vi "coutinuousPathSamplingFPGA4.vi"() -> ()   [LabVIEW 2017]
uses:
  <vilib>/rvi/Emulation/niFpgaSctlEmulationGetInTimedLoop.vi
  <vilib>/rvi/Emulation/niFpgaProcessEmulError.vi
  <vilib>/rvi/interface/RandomDataEmulation/niFpgaRandomDataHandleErrors.vi
  <vilib>/rvi/Emulation/niFpgaGetClockAttributes.vi
  <vilib>/rvi/Emulation/niFpgaEmulationReportErrorSimple.vi
  <vilib>/rvi/eio/common/nirviEmuTemplateMethod_errors.vi
  <vilib>/rvi/Emulation/niFpgaCriticalErrorInLSC.vi
  <vilib>/rvi/DataTransferAndStorage/Container/XNode/niFpgaContainer.xnode
  <vilib>/rvi/interface/RandomDataEmulation/nirviRandomDataFpgaReadWriteTemplate.vi
  <vilib>/eio/EIONode/EIONode.xnode
panel:
  out "y_image_pos_final":u16
  out "x_image_pos_final":u16
  in  "pixel distance":u16
  out "ToRead":u32
  out "increment_x_move":fxp<+/-,55,4>=0.01171875
  out "increment_y_move":fxp<+/-,55,4>=0.01171875
  out "x_FinalPos":fxp<+/-,50,5>
  out "y_FinalPos":fxp<+/-,50,5>
  in  "muPathUpdate Clock (uSec)":fxp<+,32,32>=2400.0
  in  "deflection threshold":fxp<+/-,20,5>=0.0050048828125
  in  "x threshold":fxp<+/-,20,5>=0.0050048828125
  in  "y threshold":fxp<+/-,20,5>=0.0050048828125
  in  "z threshold":fxp<+/-,20,5>=0.0050048828125
  in  "Stage Clock (uSec)":fxp<+,32,32>=500.0
  in  "pixel segment":u32
  out "SettleCheckBuffer":u16=25
  out "a tor buffer":fxp<+,17,1>[](array[numeric])=[1.9999847412109375, 1.9999847412109375, 1.9999847412109375, 1.9999847412109375, 1.9999847412109375, 1.9999847412109375, 1.9999847412109375, 1.9999847412109375, 1.9999847412109375, 1.9999847412109375, 1.9999847412109375, 1.9999847412109375, 1.9999847412109375, 1.9999847412109375, 1.9999847412109375, 1.9999847412109375, 1.9999847412109375, 1.9999847412109375, 1.9999847412109375, 1.9999847412109375, 1.9999847412109375, 1.9999847412109375, 1.9999847412109375, 1.9999847412109375, 1.9999847412109375]
  out "b tor buffer":fxp<+,17,1>[](array[numeric])=[1.9999847412109375, 1.9999847412109375, 1.9999847412109375, 1.9999847412109375, 1.9999847412109375, 1.9999847412109375, 1.9999847412109375, 1.9999847412109375, 1.9999847412109375, 1.9999847412109375, 1.9999847412109375, 1.9999847412109375, 1.9999847412109375, 1.9999847412109375, 1.9999847412109375, 1.9999847412109375, 1.9999847412109375, 1.9999847412109375, 1.9999847412109375, 1.9999847412109375, 1.9999847412109375, 1.9999847412109375, 1.9999847412109375, 1.9999847412109375, 1.9999847412109375]
  in  "deflection control":T1={"SetPoint (V)"=0.0, "scanning I"=0.03125, "scanning P"=0.0498046875, "Initial I (V)"=0.0, "Upper Limit (V)"=8.0, "Lower Limit (V)"=-8.0}
  out "deflection sensor":fxp<+/-,20,5>=-0.271331787109375
  out "zControlMode":bool
  in  "Z Clock (uSec)":fxp<+,32,32>=10.0
  out "stageIndicator":u8=1
  in  "z control":T2={"SetPoint (V)"=-0.19999980926513672, "I"=0.03125, "P"=0.0498046875, "Initial I (V)"=0.0, "Upper Limit (V)"=8.0, "Lower Limit (V)"=-8.0}
  out "signalToRecord":bool
  out "z output":fxp<+/-,64,29>=-3.5890110712498426
  in  "Sampling Clock (uSec)":fxp<+,32,32>=1500.0
  out "x output":fxp<+/-,64,29>=0.00029289722442626953
  out "y output":fxp<+/-,64,29>=0.29396580904722214
  out "x sensor":fxp<+/-,20,5>
  out "y sensor":fxp<+/-,20,5>=-0.285125732421875
  in  "XY Clock (uSec)":fxp<+,32,32>=50.0
  in  "y control":T1={"SetPoint (V)"=0.0, "scanning I"=0.03125, "scanning P"=0.0498046875, "Initial I (V)"=0.0, "Upper Limit (V)"=8.0, "Lower Limit (V)"=-8.0}
  in  "x control":T1={"SetPoint (V)"=0.0, "scanning I"=0.03125, "scanning P"=0.0498046875, "Initial I (V)"=0.0, "Upper Limit (V)"=8.0, "Lower Limit (V)"=-8.0}
  out "signalToStop":bool
  out "x_pos":fxp<+/-,50,5>=0.005859375
  out "y_pos":fxp<+/-,50,5>=0.005859375
  out "increment_x":fxp<+/-,50,5>=0.01171875
  out "increment_y":fxp<+/-,50,5>=0.01171875
  in  "ImageToSample":T3={"image size_x"=256, "image size_y"=256, "sample start_x"=0.0, "sample start_y"=0.0, "sample end_x"=3.0, "sample end_y"=3.0}
  out "y_image_pos":u16
  out "x_image_pos":u16
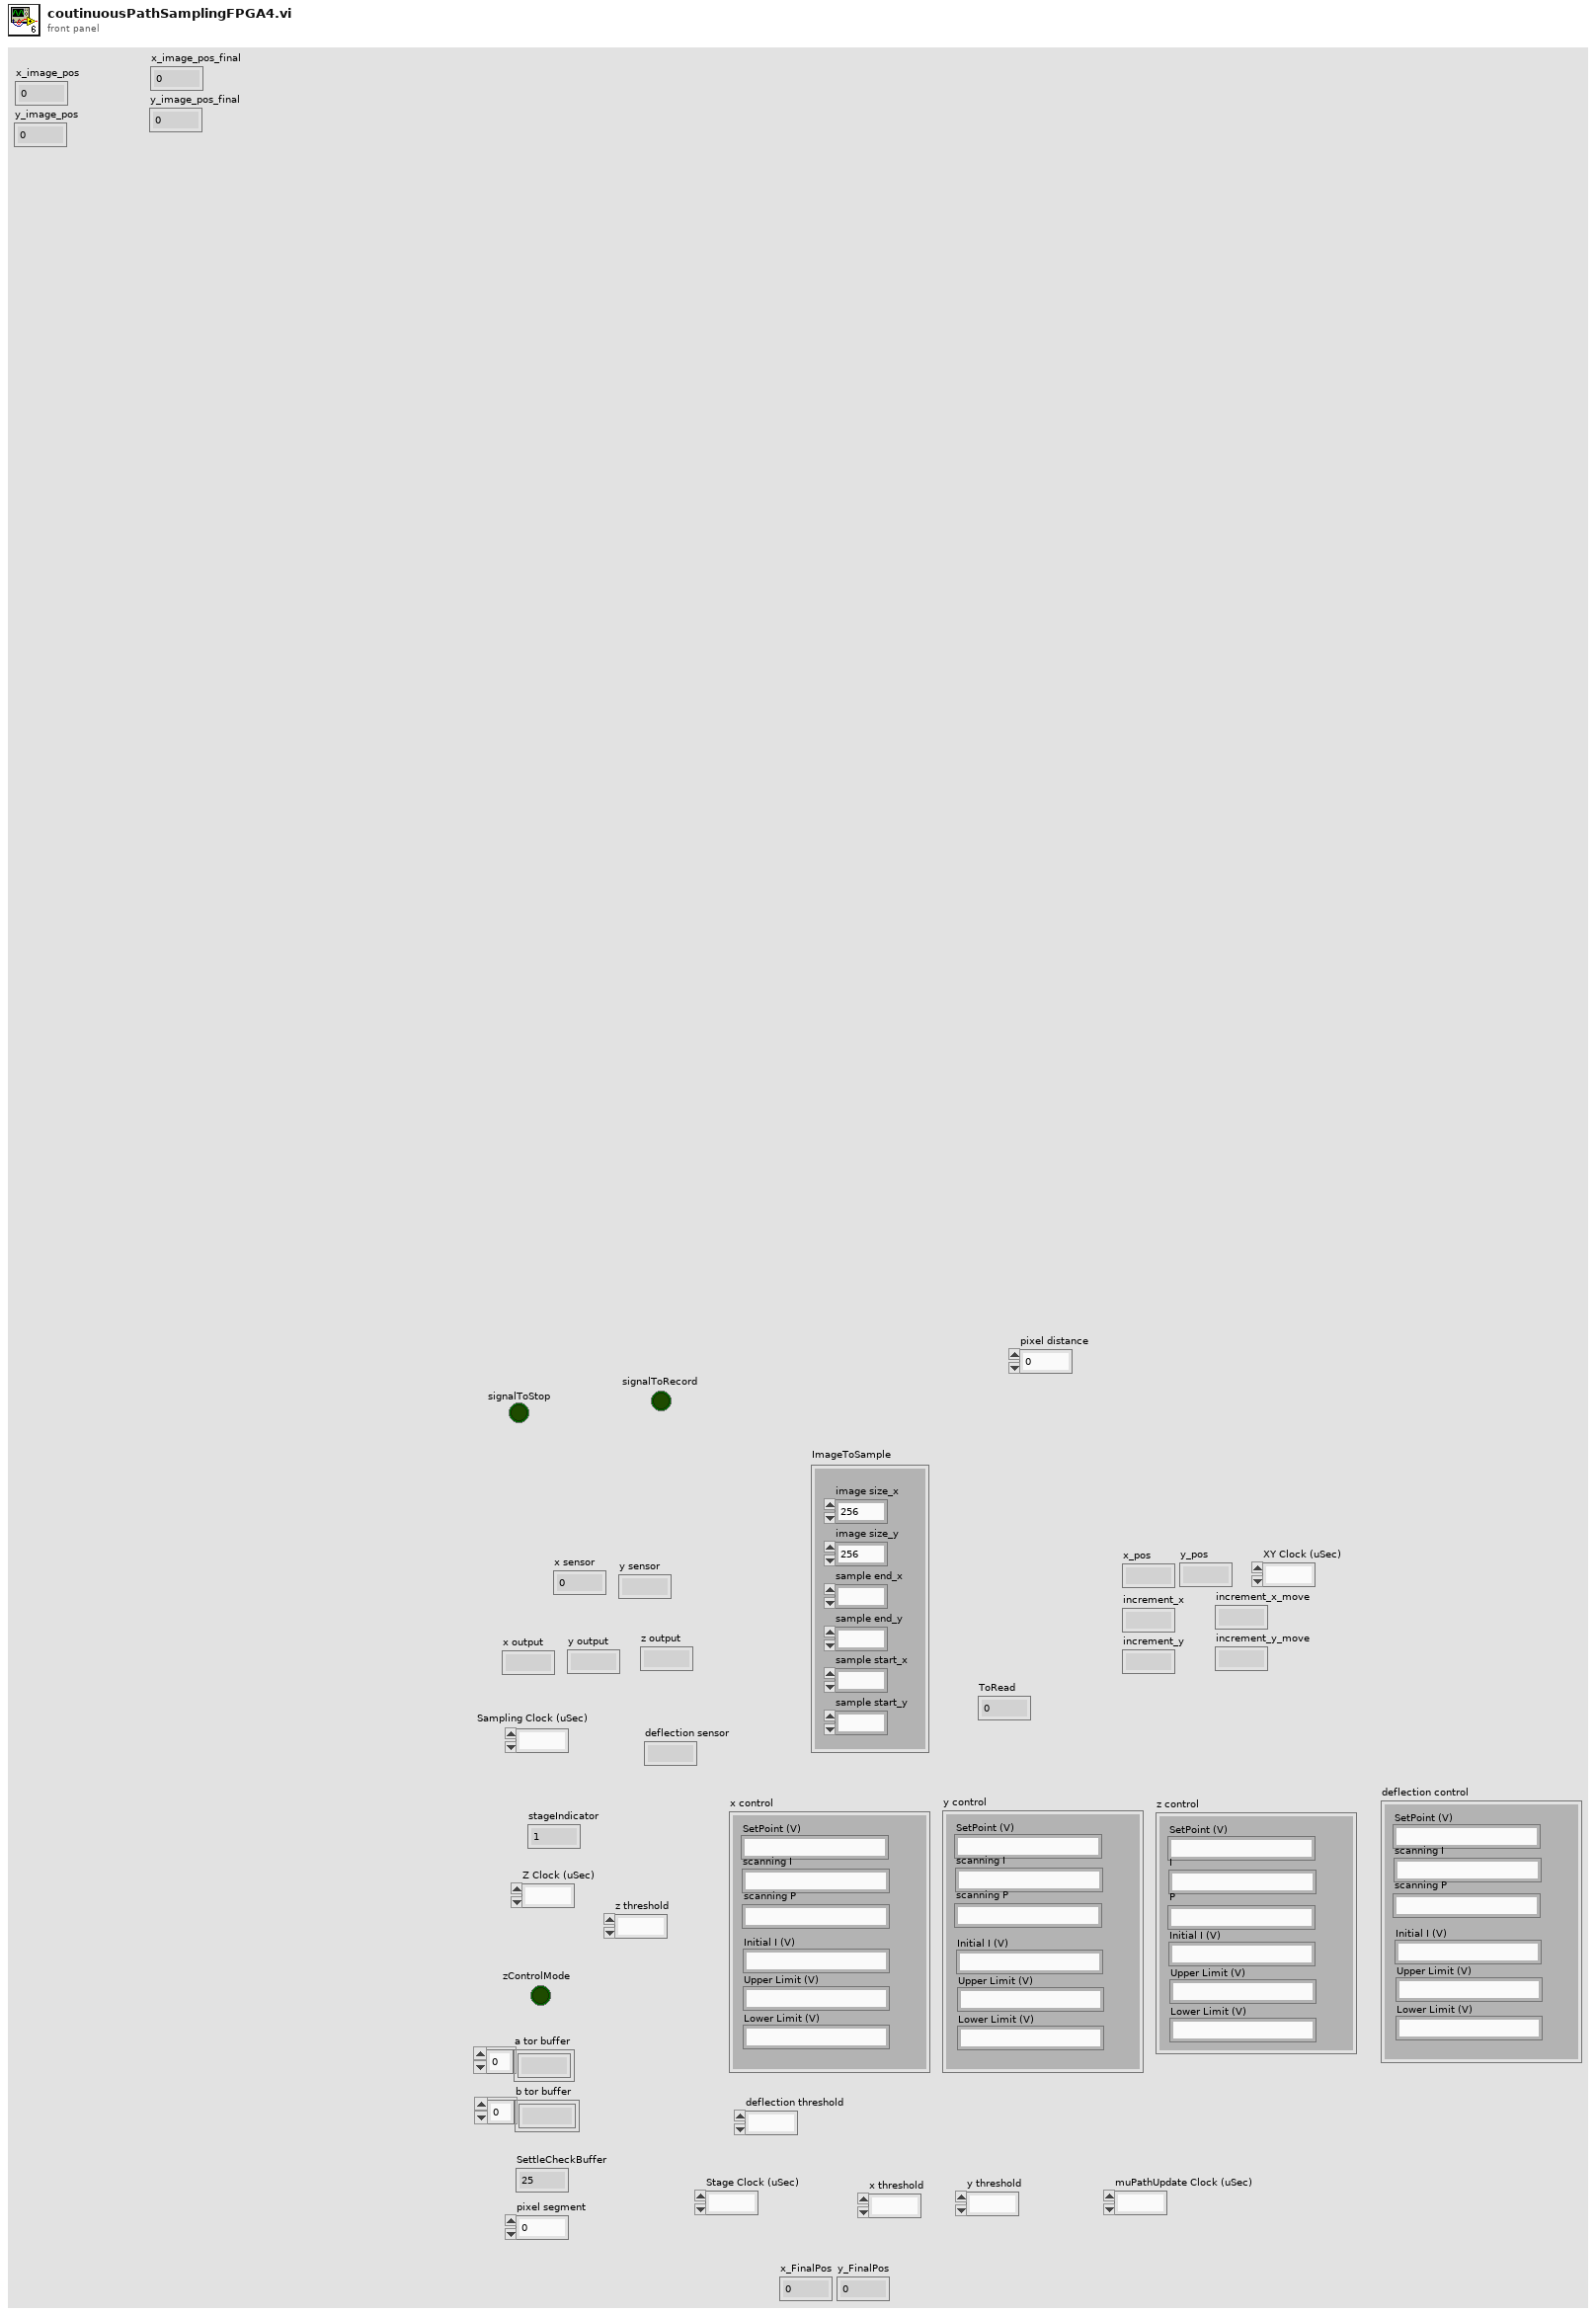
[diagram p1: front panel]
types:
  T1 = cluster{"SetPoint (V)":fxp<+/-,26,5>, "scanning I":fxp<+,21,13>, "scanning P":fxp<+,15,5>, "Initial I (V)":fxp<+/-,10,5>, "Upper Limit (V)":fxp<+/-,26,5>, "Lower Limit (V)":fxp<+/-,26,5>}
  T2 = cluster{"SetPoint (V)":fxp<+/-,26,5>, "I":fxp<+,21,13>, "P":fxp<+,15,5>, "Initial I (V)":fxp<+/-,10,5>, "Upper Limit (V)":fxp<+/-,26,5>, "Lower Limit (V)":fxp<+/-,26,5>}
  T3 = cluster{"image size_x":u16, "image size_y":u16, "sample start_x":fxp<+/-,26,5>, "sample start_y":fxp<+/-,26,5>, "sample end_x":fxp<+/-,26,5>, "sample end_y":fxp<+/-,26,5>}
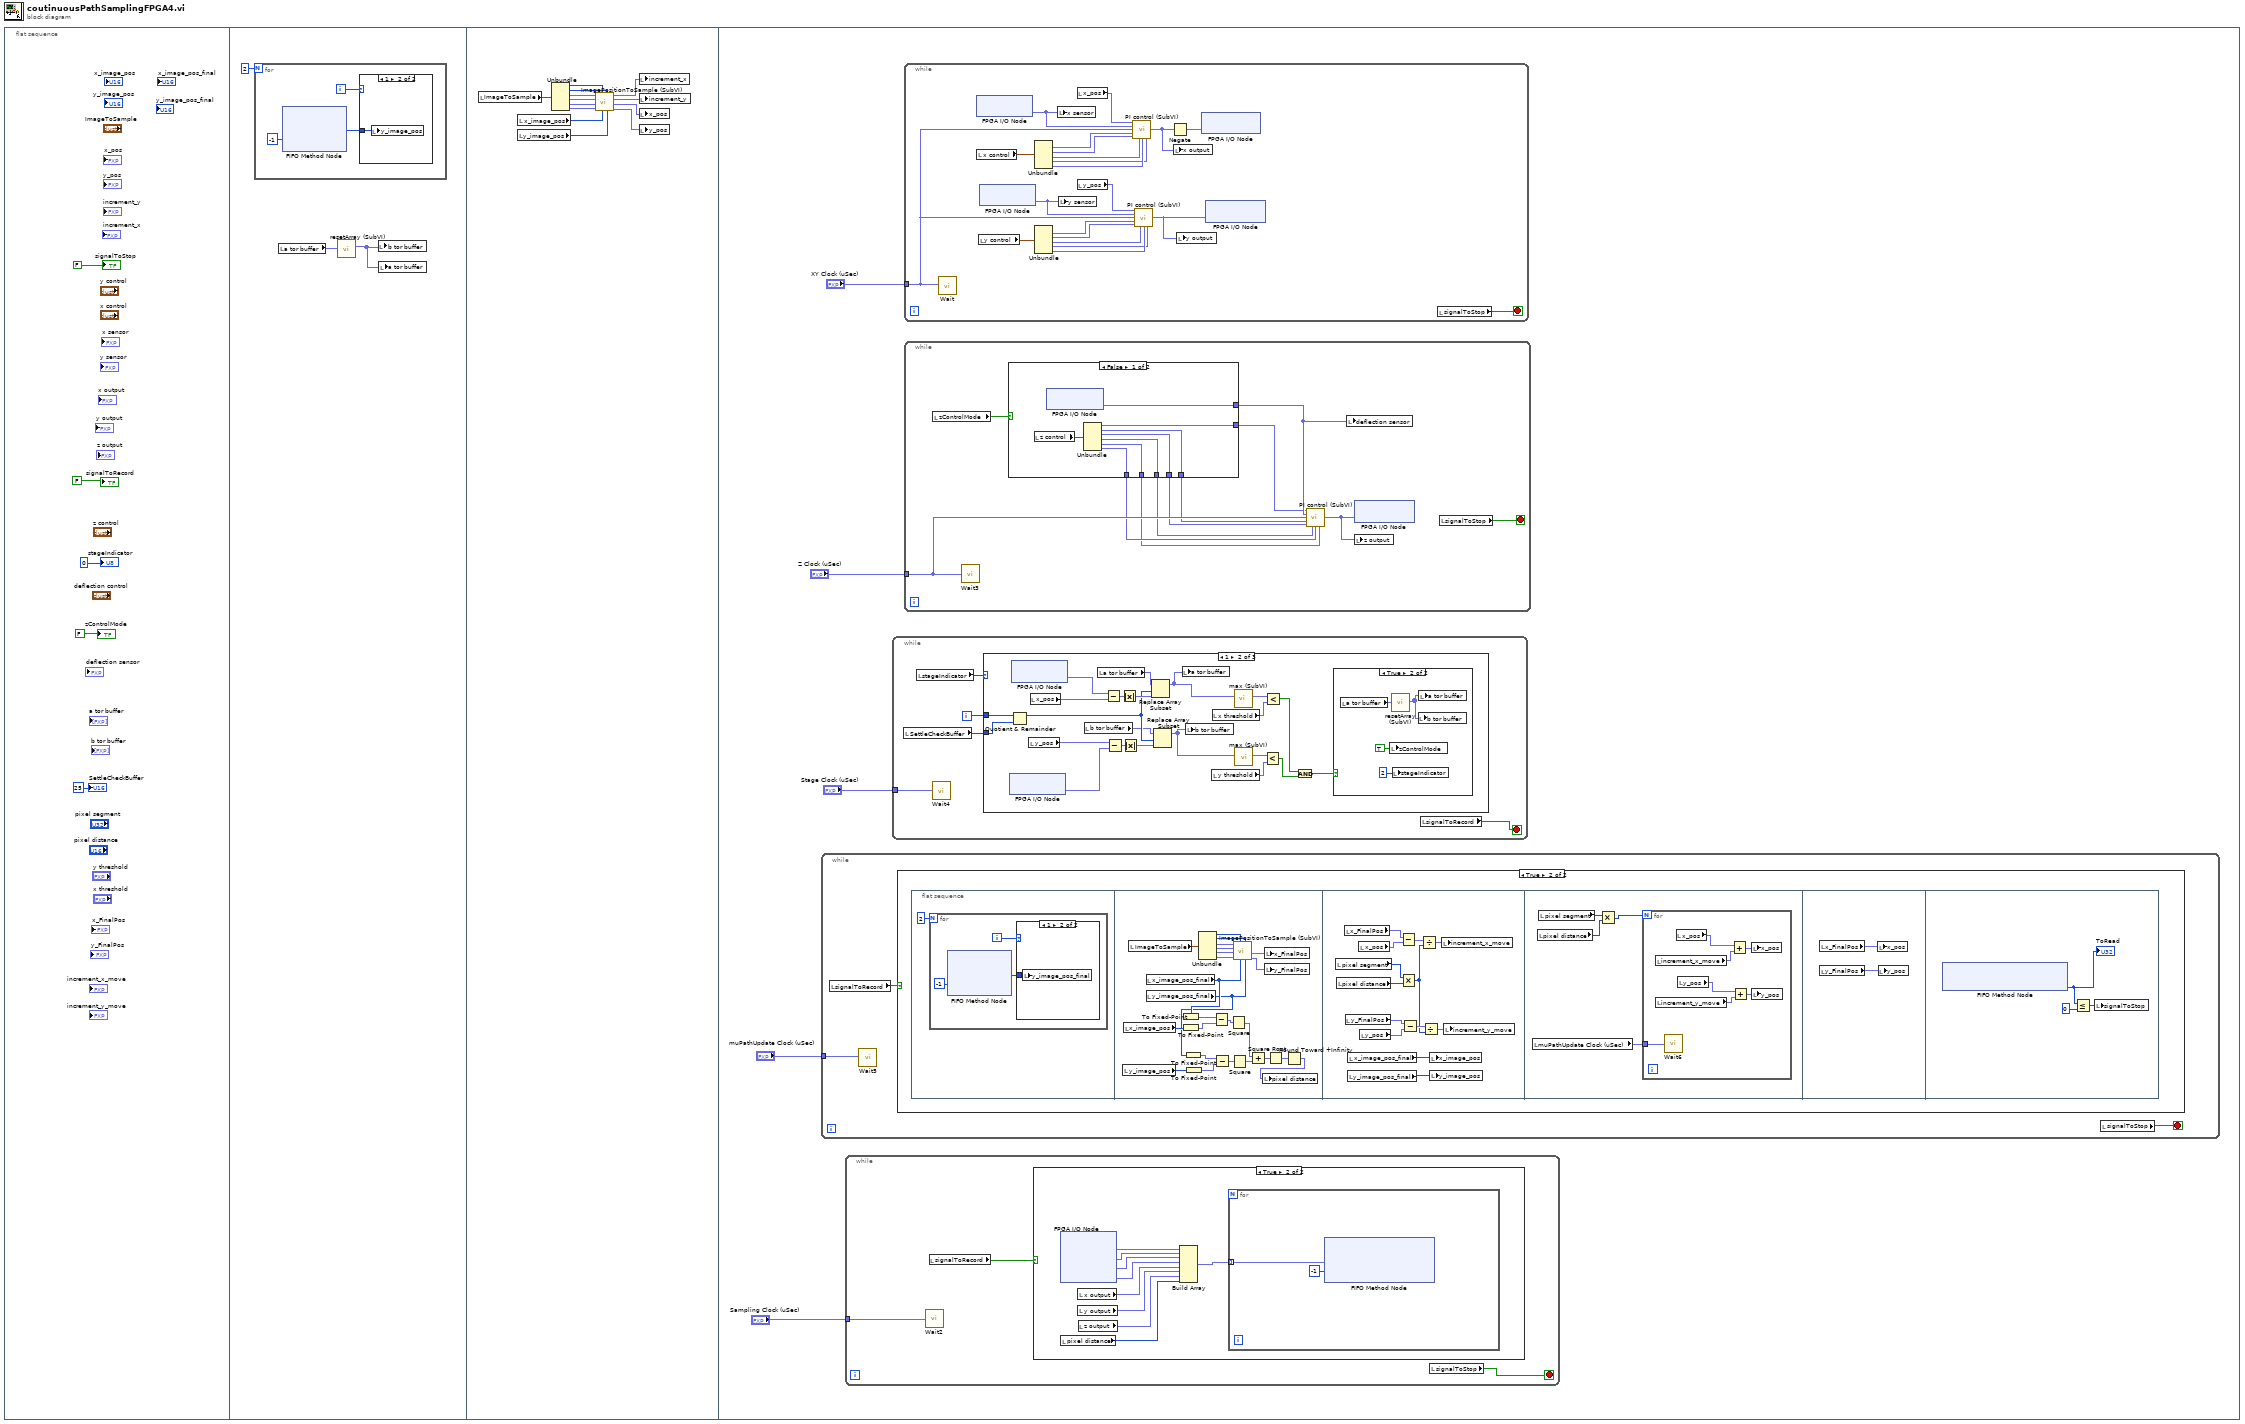
[diagram p0: block diagram]
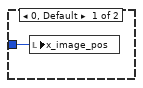
[diagram p2: hidden frame]
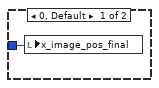
[diagram p4: hidden frame]
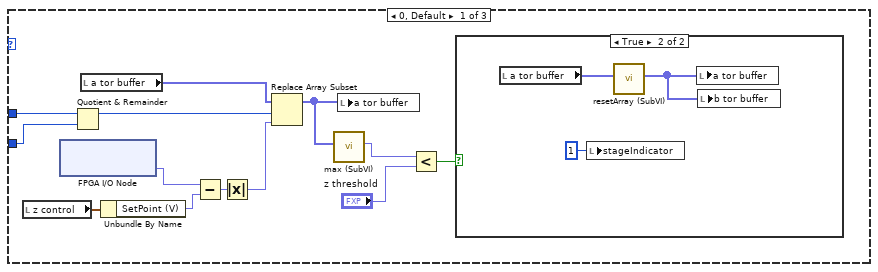
[diagram p5: hidden frame]
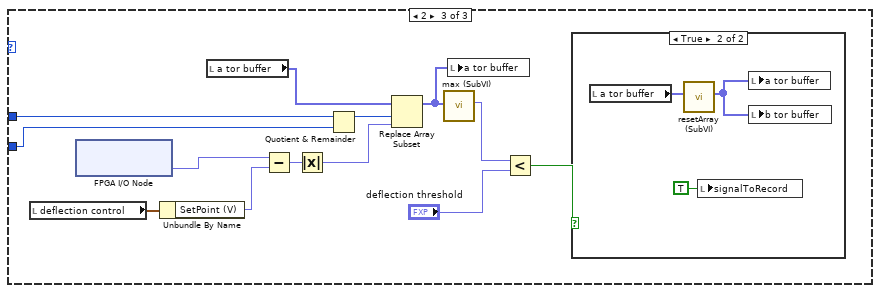
[diagram p8: hidden frame]
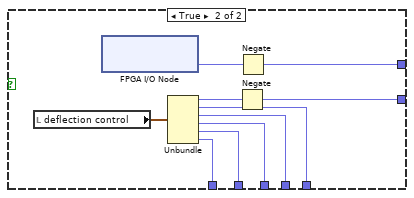
[diagram p10: hidden frame]
diagram:
  n1 = flat-sequence {
    frame #0 {
      "signalToStop" <- FALSE ("signalToStop")
      "signalToRecord" <- FALSE ("signalToRecord")
      "stageIndicator" <- u8 0 ("stageIndicator")
      "zControlMode" <- FALSE ("zControlMode")
      "SettleCheckBuffer" <- u16 25 ("SettleCheckBuffer")
    }
    frame #1 {
      n2 = for {
        N: 2 -> [_]
        i -> [w10]
        n3 = xnode ("FIFO Method Node")("Timeout"=-1) -> ("Element"=w9:u16)  [unwired: 1 in, 2 out]
        n4 = case shown="1" w10 {
          tunnel: w9 -> [w12 w13]
          frame 0, Default {
            n5 = local write "x_image_pos"(w12) -> ()
          }
          frame 1 {
            n6 = local write "y_image_pos"(w13) -> ()
          }
        }
      }
      n7 = local read "a tor buffer"() -> (w7:fxp<+,17,1>[])
      n8 = call "resetArray (SubVI).vi"("a samples in"=w7) -> ("a samples out"=w6:fxp<+/-,64,32>[])  [unwired: 10 in]
      n9 = local write "b tor buffer"(w6) -> ()
      n10 = local write "a tor buffer"(w6) -> ()
    }
    frame #2 {
      n11 = local read "ImageToSample"() -> (w26:T3)
      n12 = local read "y_image_pos"() -> (w18:u16)
      n13 = local read "x_image_pos"() -> (w19:u16)
      n14 = Unbundle(w26) -> ("image size_x"=w25:u16, "image size_y"=w24:u16, "sample start_x"=w23:fxp<+/-,26,5>, "sample start_y"=w22:fxp<+/-,26,5>, "sample end_x"=w21:fxp<+/-,26,5>, "sample end_y"=w20:fxp<+/-,26,5>)
      n15 = call "ImagePositionToSample (SubVI).vi"("image_y"=w18, "image size_y"=w24, "image_x"=w19, "image size_x"=w25, "sample end_y"=w20, "sample end_x"=w21, "sample start_y"=w22, "sample start_x"=w23) -> ("sample_y"=w14:fxp<+/-,26,5>, "sample_x"=w15:fxp<+/-,26,5>, "increment_y"=w16:fxp<+/-,26,5>, "increment_x"=w17:fxp<+/-,26,5>)
      n16 = local write "increment_x"(w17) -> ()
      n17 = local write "increment_y"(w16) -> ()
      n18 = local write "x_pos"(w15) -> ()
      n19 = local write "y_pos"(w14) -> ()
    }
    frame #3 {
      n20 = while {
        tunnel: "muPathUpdate Clock (uSec)" -> [w33]
        stop <- w34 stop-if-true
        n21 = local read "signalToRecord"() -> (w32:bool)
        n22 = call "Wait5"("Count(uSec)"=w33) -> ()  [unwired: 1 out]
        n23 = case shown="True" w32 {
          frame False {
          }
          frame True {
            n24 = flat-sequence {
              frame #0 {
                n25 = for {
                  N: 2 -> [_]
                  i -> [w37]
                  n26 = xnode ("FIFO Method Node")("Timeout"=-1) -> ("Element"=w36:u16)  [unwired: 1 in, 2 out]
                  n27 = case shown="1" w37 {
                    tunnel: w36 -> [w39 w40]
                    frame 0, Default {
                      n28 = local write "x_image_pos_final"(w39) -> ()
                    }
                    frame 1 {
                      n29 = local write "y_image_pos_final"(w40) -> ()
                    }
                  }
                }
              }
              frame #1 {
                n30 = local read "y_image_pos"() -> (w46:u16)
                n31 = local read "x_image_pos"() -> (w47:u16)
                n32 = local read "ImageToSample"() -> (w64:T3)
                n33 = local read "x_image_pos_final"() -> (w50:u16)
                n34 = local read "y_image_pos_final"() -> (w43:u16)
                n35 = To Fixed-Point(number=w50) -> (fixed-point=w49:fxp<+,16,16>)  [unwired: 1 in]
                n36 = To Fixed-Point(number=w47) -> (fixed-point=w48:fxp<+,16,16>)  [unwired: 1 in]
                n37 = To Fixed-Point(number=w43) -> (fixed-point=w44:fxp<+,16,16>)  [unwired: 1 in]
                n38 = To Fixed-Point(number=w46) -> (fixed-point=w45:fxp<+,16,16>)  [unwired: 1 in]
                n39 = Unbundle(w64) -> ("image size_x"=w63:u16, "image size_y"=w62:u16, "sample start_x"=w61:fxp<+/-,26,5>, "sample start_y"=w60:fxp<+/-,26,5>, "sample end_x"=w59:fxp<+/-,26,5>, "sample end_y"=w58:fxp<+/-,26,5>)
                n40 = Subtract(x=w49, y=w48) -> (x-y=w52:fxp<+/-,17,17>)
                n41 = Subtract(x=w44, y=w45) -> (x-y=w51:fxp<+/-,17,17>)
                n42 = Square(x=w52) -> (x^2=w54:fxp<+,32,32>)
                n43 = Square(x=w51) -> (x^2=w55:fxp<+,32,32>)
                n44 = call "ImagePositionToSample (SubVI).vi"("image_y"=w43, "image size_y"=w62, "image_x"=w50, "image size_x"=w63, "sample end_y"=w58, "sample end_x"=w59, "sample start_y"=w60, "sample start_x"=w61) -> ("sample_y"=w56:fxp<+/-,26,5>, "sample_x"=w57:fxp<+/-,26,5>)  [unwired: 2 out]
                n45 = Add(x=w54, y=w55) -> (x+y=w53:fxp<+,33,33>)
                n46 = local write "x_FinalPos"(w57) -> ()
                n47 = local write "y_FinalPos"(w56) -> ()
                n48 = Square Root(x=w53) -> (sqrt(x)=w42:fxp<+,36,17>)
                n49 = Round Toward +Infinity(x=w42) -> (ceil(x): smallest int >= x=w41:fxp<+,17,17>)
                n50 = local write "pixel distance"(w41) -> ()
              }
              frame #2 {
                n51 = local read "pixel segment"() -> (w68:u32)
                n52 = local read "pixel distance"() -> (w67:u16)
                n53 = local read "x_FinalPos"() -> (w77:fxp<+/-,50,5>)
                n54 = local read "y_FinalPos"() -> (w71:fxp<+/-,50,5>)
                n55 = local read "y_image_pos_final"() -> (w65:u16)
                n56 = local read "x_image_pos_final"() -> (w66:u16)
                n57 = local read "x_pos"() -> (w76:fxp<+/-,50,5>)
                n58 = local read "y_pos"() -> (w70:fxp<+/-,50,5>)
                n59 = Subtract(x=w77, y=w76) -> (x-y=w75:fxp<+/-,51,6>)
                n60 = Multiply(x=w68, y=w67) -> (x*y=w69:u32)
                n61 = Subtract(x=w71, y=w70) -> (x-y=w73:fxp<+/-,51,6>)
                n62 = Divide(x=w75, y=w69) -> (x/y=w74:fxp<+/-,64,6>)
                n63 = Divide(x=w73, y=w69) -> (x/y=w72:fxp<+/-,64,6>)
                n64 = local write "x_image_pos"(w66) -> ()
                n65 = local write "y_image_pos"(w65) -> ()
                n66 = local write "increment_x_move"(w74) -> ()
                n67 = local write "increment_y_move"(w72) -> ()
              }
              frame #3 {
                n68 = local read "muPathUpdate Clock (uSec)"() -> (w81:fxp<+,32,32>)
                n69 = local read "pixel distance"() -> (w78:u16)
                n70 = local read "pixel segment"() -> (w80:u32)
                n71 = Multiply(x=w80, y=w78) -> (x*y=w79:u32)
                n72 = for {
                  N: w79 -> [_]
                  tunnel: w81 -> [w88]
                  n73 = local read "increment_x_move"() -> (w86:fxp<+/-,55,4>)
                  n74 = local read "increment_y_move"() -> (w83:fxp<+/-,55,4>)
                  n75 = call "Wait6"("Count(uSec)"=w88) -> ()  [unwired: 1 out]
                  n76 = local read "x_pos"() -> (w87:fxp<+/-,50,5>)
                  n77 = local read "y_pos"() -> (w84:fxp<+/-,50,5>)
                  n78 = Add(x=w87, y=w86) -> (x+y=w85:fxp<+/-,57,6>)
                  n79 = Add(x=w84, y=w83) -> (x+y=w82:fxp<+/-,57,6>)
                  n80 = local write "x_pos"(w85) -> ()
                  n81 = local write "y_pos"(w82) -> ()
                }
              }
              frame #4 {
                n82 = local read "x_FinalPos"() -> (w90:fxp<+/-,50,5>)
                n83 = local read "y_FinalPos"() -> (w89:fxp<+/-,50,5>)
                n84 = local write "x_pos"(w90) -> ()
                n85 = local write "y_pos"(w89) -> ()
              }
              frame #5 {
                n86 = xnode ("FIFO Method Node")() -> ("Number of Elements to Read"=w91:u32)  [unwired: 1 in, 1 out]
                "ToRead" <- w91
                n87 = Less Or Equal?(x=w91, y=u32 0) -> (x <= y?=w92:bool)
                n88 = local write "signalToStop"(w92) -> ()
              }
            }
          }
        }
        n89 = local read "signalToStop"() -> (w34:bool)
      }
      n90 = while {
        tunnel: "Sampling Clock (uSec)" -> [w188]
        stop <- w187 stop-if-true
        n91 = call "Wait2"("Count(uSec)"=w188) -> ()  [unwired: 1 out]
        n92 = local read "signalToRecord"() -> (w186:bool)
        n93 = case shown="True" w186 {
          frame False {
          }
          frame True {
            n94 = xnode "FPGA I/O Node"() -> ("Mod1/AI0"=w197:fxp<+/-,20,5>, "Mod1/AI1"=w196:fxp<+/-,20,5>, "Mod1/AI2"=w195:fxp<+/-,20,5>, "Mod1/AI3"=w194:fxp<+/-,20,5>)  [unwired: 4 in, 4 out]
            n95 = local read "pixel distance"() -> (w189:u16)
            n96 = local read "x output"() -> (w193:fxp<+/-,64,29>)
            n97 = local read "y output"() -> (w192:fxp<+/-,64,29>)
            n98 = local read "z output"() -> (w191:fxp<+/-,64,29>)
            n99 = Build Array(w197, w196, w195, w194, w193, w192, w191, w189) -> (w190:fxp<+/-,64,29>[])
            n100 = for {
              tunnel: w190 -> [w199] mode=indexing
              n101 = xnode ("FIFO Method Node")("Element"=w199, "Timeout"=-1) -> ()  [unwired: 1 in, 2 out]
            }
          }
        }
        n102 = local read "signalToStop"() -> (w187:bool)
      }
      n103 = while {
        tunnel: "Stage Clock (uSec)" -> [w98]
        i -> [w96]
        stop <- w94 stop-if-true
        n104 = local read "SettleCheckBuffer"() -> (w95:u16)
        n105 = local read "stageIndicator"() -> (w97:u8)
        n106 = call "Wait4"("Count(uSec)"=w98) -> ()  [unwired: 1 out]
        n107 = case shown="1" w97 {
          tunnel: w96 -> [w111 w136 w153]
          tunnel: w95 -> [w110 w135 w152]
          frame 0, Default {
            n108 = local read "z control"() -> (w104:T2)
            n109 = xnode "FPGA I/O Node"() -> ("Mod1/AI2"=w106:fxp<+/-,20,5>)  [unwired: 1 in, 1 out]
            n110 = Quotient & Remainder(x=w111, y=w110) -> (x-y*floor(x/y)=w109:i32)  [unwired: 1 out]
            n111 = local read "a tor buffer"() -> (w105:fxp<+,17,1>[])
            n112 = Unbundle By Name(w104) -> ("SetPoint (V)"=w103:fxp<+/-,26,5>)
            n113 = Subtract(x=w106, y=w103) -> (x-y=w108:fxp<+/-,27,6>)
            n114 = Absolute Value(x=w108) -> (abs(x)=w107:fxp<+,26,5>)
            n115 = Replace Array Subset(array=w105, new element=w107, index=w109) -> (w102:fxp<+,17,1>[])
            n116 = call "max (SubVI).vi"("initialized array"=w102) -> ("y"=w101:fxp<+/-,64,32>)  [unwired: 10 in]
            n117 = local write "a tor buffer"(w102) -> ()
            n118 = Less?(x=w101, y="z threshold") -> (x < y?=w99:bool)
            n119 = case shown="True" w99 {
              frame False {
              }
              frame True {
                n120 = local read "a tor buffer"() -> (w114:fxp<+,17,1>[])
                n121 = local write "stageIndicator"(u8 1 ("stageIndicator")) -> ()
                n122 = call "resetArray (SubVI).vi"("a samples in"=w114) -> ("a samples out"=w113:fxp<+/-,64,32>[])  [unwired: 10 in]
                n123 = local write "a tor buffer"(w113) -> ()
                n124 = local write "b tor buffer"(w113) -> ()
              }
            }
          }
          frame 1 {
            n125 = xnode "FPGA I/O Node"() -> ("Mod1/AI1"=w117:fxp<+/-,20,5>)  [unwired: 1 in, 1 out]
            n126 = Quotient & Remainder(x=w136, y=w135) -> (x-y*floor(x/y)=w127:i32)  [unwired: 1 out]
            n127 = xnode "FPGA I/O Node"() -> ("Mod1/AI0"=w118:fxp<+/-,20,5>)  [unwired: 1 in, 1 out]
            n128 = local read "y_pos"() -> (w115:fxp<+/-,50,5>)
            n129 = local read "x_pos"() -> (w116:fxp<+/-,50,5>)
            n130 = local read "b tor buffer"() -> (w125:fxp<+,17,1>[])
            n131 = local read "a tor buffer"() -> (w126:fxp<+,17,1>[])
            n132 = Subtract(x=w118, y=w116) -> (x-y=w131:fxp<+/-,51,6>)
            n133 = Subtract(x=w115, y=w117) -> (x-y=w129:fxp<+/-,51,6>)
            n134 = Absolute Value(x=w131) -> (abs(x)=w130:fxp<+,50,5>)
            n135 = Absolute Value(x=w129) -> (abs(x)=w128:fxp<+,50,5>)
            n136 = Replace Array Subset(array=w126, new element=w130, index=w127) -> (w124:fxp<+,17,1>[])
            n137 = Replace Array Subset(array=w125, new element=w128, index=w127) -> (w123:fxp<+,17,1>[])
            n138 = local write "a tor buffer"(w124) -> ()
            n139 = local write "b tor buffer"(w123) -> ()
            n140 = local read "y threshold"() -> (w119:fxp<+/-,20,5>)
            n141 = local read "x threshold"() -> (w121:fxp<+/-,20,5>)
            n142 = call "max (SubVI).vi"("initialized array"=w124) -> ("y"=w122:fxp<+/-,64,32>)  [unwired: 10 in]
            n143 = call "max (SubVI).vi"("initialized array"=w123) -> ("y"=w120:fxp<+/-,64,32>)  [unwired: 10 in]
            n144 = Less?(x=w120, y=w119) -> (x < y?=w133:bool)
            n145 = Less?(x=w122, y=w121) -> (x < y?=w134:bool)
            n146 = And(x=w134, y=w133) -> (x .and. y?=w132:bool)
            n147 = case shown="True" w132 {
              frame False {
              }
              frame True {
                n148 = local read "a tor buffer"() -> (w139:fxp<+,17,1>[])
                n149 = local write "zControlMode"(TRUE ("zControlMode")) -> ()
                n150 = call "resetArray (SubVI).vi"("a samples in"=w139) -> ("a samples out"=w138:fxp<+/-,64,32>[])  [unwired: 10 in]
                n151 = local write "stageIndicator"(u8 2 ("stageIndicator")) -> ()
                n152 = local write "b tor buffer"(w138) -> ()
                n153 = local write "a tor buffer"(w138) -> ()
              }
            }
          }
          frame 2 {
            n154 = local read "deflection control"() -> (w149:T1)
            n155 = xnode "FPGA I/O Node"() -> ("Mod1/AI3"=w147:fxp<+/-,20,5>)  [unwired: 1 in, 1 out]
            n156 = Unbundle By Name(w149) -> ("SetPoint (V)"=w148:fxp<+/-,26,5>)
            n157 = local read "a tor buffer"() -> (w143:fxp<+,17,1>[])
            n158 = Subtract(x=w147, y=w148) -> (x-y=w151:fxp<+/-,27,6>)
            n159 = Absolute Value(x=w151) -> (abs(x)=w146:fxp<+,26,5>)
            n160 = Quotient & Remainder(x=w153, y=w152) -> (x-y*floor(x/y)=w150:i32)  [unwired: 1 out]
            n161 = Replace Array Subset(array=w143, new element=w146, index=w150) -> (w142:fxp<+,17,1>[])
            n162 = call "max (SubVI).vi"("initialized array"=w142) -> ("y"=w145:fxp<+/-,64,32>)  [unwired: 10 in]
            n163 = local write "a tor buffer"(w142) -> ()
            n164 = Less?(x=w145, y="deflection threshold") -> (x < y?=w141:bool)
            n165 = case shown="True" w141 {
              frame False {
              }
              frame True {
                n166 = local read "a tor buffer"() -> (w156:fxp<+,17,1>[])
                n167 = call "resetArray (SubVI).vi"("a samples in"=w156) -> ("a samples out"=w155:fxp<+/-,64,32>[])  [unwired: 10 in]
                n168 = local write "signalToRecord"(TRUE ("signalToRecord")) -> ()
                n169 = local write "a tor buffer"(w155) -> ()
                n170 = local write "b tor buffer"(w155) -> ()
              }
            }
          }
        }
        n171 = local read "signalToRecord"() -> (w94:bool)
      }
      n172 = while {
        tunnel: "XY Clock (uSec)" -> [w206]
        stop <- w220 stop-if-true
        n173 = call "Wait"("Count(uSec)"=w206) -> ()  [unwired: 1 out]
        n174 = xnode "FPGA I/O Node"() -> ("Mod1/AI0"=w217:fxp<+/-,20,5>)  [unwired: 1 in, 1 out]
        n175 = local read "x control"() -> (w219:T1)
        n176 = local read "y control"() -> (w207:T1)
        n177 = xnode "FPGA I/O Node"() -> ("Mod1/AI1"=w208:fxp<+/-,20,5>)  [unwired: 1 in, 1 out]
        n178 = Unbundle(w219) -> ("scanning I"=w216:fxp<+,21,13>, "scanning P"=w215:fxp<+,15,5>, "Initial I (V)"=w214:fxp<+/-,10,5>, "Upper Limit (V)"=w212:fxp<+/-,26,5>, "Lower Limit (V)"=w213:fxp<+/-,26,5>)  [unwired: 1 out]
        n179 = Unbundle(w207) -> ("scanning I"=w205:fxp<+,21,13>, "scanning P"=w204:fxp<+,15,5>, "Initial I (V)"=w203:fxp<+/-,10,5>, "Upper Limit (V)"=w201:fxp<+/-,26,5>, "Lower Limit (V)"=w202:fxp<+/-,26,5>)  [unwired: 1 out]
        n180 = local write "x sensor"(w217) -> ()
        n181 = local write "y sensor"(w208) -> ()
        n182 = local read "x_pos"() -> (w218:fxp<+/-,50,5>)
        n183 = local read "y_pos"() -> (w209:fxp<+/-,50,5>)
        n184 = call "PI control (SubVI).vi"("SetPoint"=w218, "Feedback"=w217, "Clock"=w206, "I"=w216, "P"=w215, "Initial I"=w214, "Lower Limit"=w213, "Upper Limit in"=w212) -> ("Output"=w211:fxp<+/-,20,5>)  [unwired: 7 in]
        n185 = call "PI control (SubVI).vi"("SetPoint"=w209, "Feedback"=w208, "Clock"=w206, "I"=w205, "P"=w204, "Initial I"=w203, "Lower Limit"=w202, "Upper Limit in"=w201) -> ("Output"=w200:fxp<+/-,20,5>)  [unwired: 7 in]
        n186 = Negate(x=w211) -> (-x=w210:fxp<+/-,21,6>)
        n187 = local write "x output"(w211) -> ()
        n188 = local write "y output"(w200) -> ()
        n189 = xnode "FPGA I/O Node"("Mod8/AO0"=w210) -> ()  [unwired: 1 in, 1 out]
        n190 = xnode "FPGA I/O Node"("Mod8/AO1"=w200) -> ()  [unwired: 1 in, 1 out]
        n191 = local read "signalToStop"() -> (w220:bool)
      }
      n192 = while {
        tunnel: "Z Clock (uSec)" -> [w162]
        stop <- w167 stop-if-true
        n193 = local read "zControlMode"() -> (w166:bool)
        n194 = call "Wait3"("Count(uSec)"=w162) -> ()  [unwired: 1 out]
        n195 = case shown="False" w166 {
          tunnel: [w174 w183] -> w164
          tunnel: [w173 w181] -> w163
          tunnel: [w172 w180] -> w161
          tunnel: [w171 w179] -> w160
          tunnel: [w170 w178] -> w159
          tunnel: [w169 w177] -> w158
          tunnel: [w168 w176] -> w157
          frame False {
            n196 = local read "z control"() -> (w175:T2)
            n197 = xnode "FPGA I/O Node"() -> ("Mod1/AI2"=w174:fxp<+/-,20,5>)  [unwired: 1 in, 1 out]
            n198 = Unbundle(w175) -> ("SetPoint (V)"=w173:fxp<+/-,26,5>, "I"=w172:fxp<+,21,13>, "P"=w171:fxp<+,15,5>, "Initial I (V)"=w170:fxp<+/-,10,5>, "Upper Limit (V)"=w168:fxp<+/-,26,5>, "Lower Limit (V)"=w169:fxp<+/-,26,5>)
          }
          frame True {
            n199 = local read "deflection control"() -> (w185:T1)
            n200 = xnode "FPGA I/O Node"() -> ("Mod1/AI3"=w184:fxp<+/-,20,5>)  [unwired: 1 in, 1 out]
            n201 = Unbundle(w185) -> ("SetPoint (V)"=w182:fxp<+/-,26,5>, "scanning I"=w180:fxp<+,21,13>, "scanning P"=w179:fxp<+,15,5>, "Initial I (V)"=w178:fxp<+/-,10,5>, "Upper Limit (V)"=w176:fxp<+/-,26,5>, "Lower Limit (V)"=w177:fxp<+/-,26,5>)
            n202 = Negate(x=w182) -> (-x=w181:fxp<+/-,27,6>)
            n203 = Negate(x=w184) -> (-x=w183:fxp<+/-,21,6>)
          }
        }
        n204 = call "PI control (SubVI).vi"("SetPoint"=w163, "Feedback"=w164, "Clock"=w162, "I"=w161, "P"=w160, "Initial I"=w159, "Lower Limit"=w158, "Upper Limit in"=w157) -> ("Output"=w165:fxp<+/-,20,5>)  [unwired: 7 in]
        n205 = local write "deflection sensor"(w164) -> ()
        n206 = xnode "FPGA I/O Node"("Mod8/AO2"=w165) -> ()  [unwired: 1 in, 1 out]
        n207 = local write "z output"(w165) -> ()
        n208 = local read "signalToStop"() -> (w167:bool)
      }
    }
  }
